vi "SCMP - darkflat.vi"(8 "error in (no error)":errorcluster, 10 "Dark/Flat":bool, 11 "Image Data Cluser":T1) -> (0 "error out":errorcluster, 2 "Raw Image Data2":u16[][](array[numeric]), 3 "Raw Image Data1":u16[][](array[numeric]), 4 "Y scale":i32, 6 "Image Data":u32[][](array[numeric]))   [LabVIEW 2014]
panel:
  out "dark/flat image":u32[][](graph)
  out "raw image":u32[][](graph)
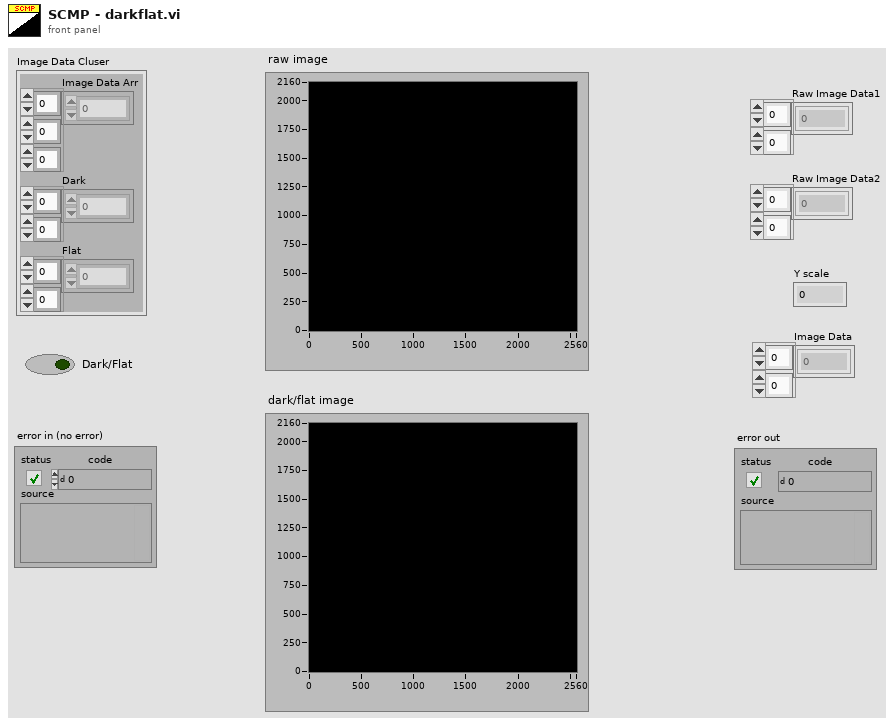
[diagram p1: front panel]
types:
  T1 = cluster{"Image Data Arr":u32[][][], "Dark":u32[][], "Flat":u32[][]}
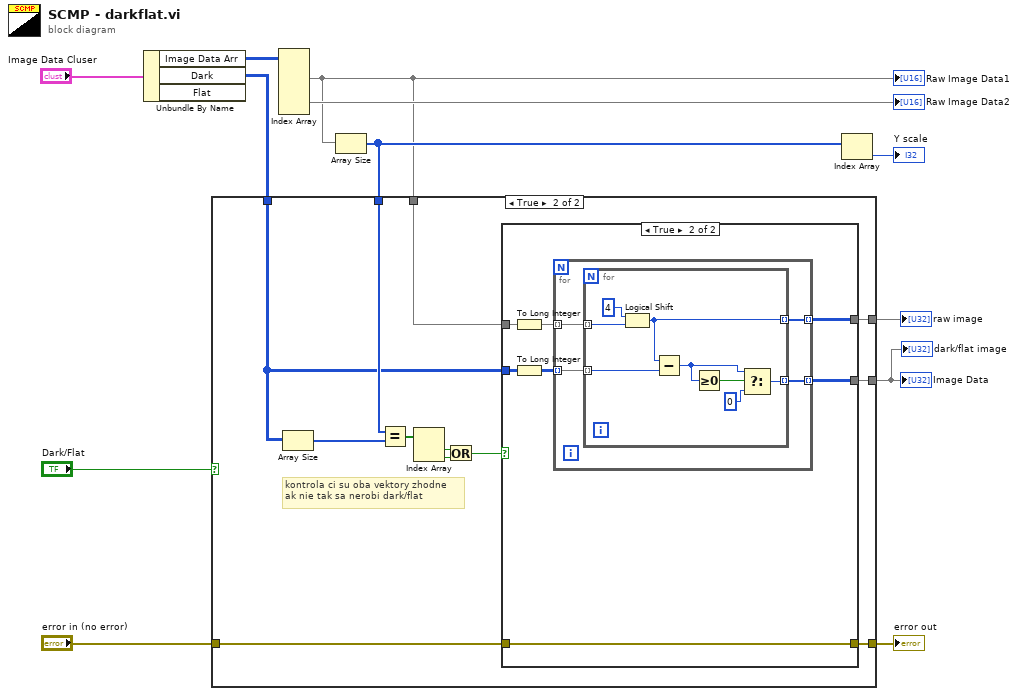
[diagram p0: block diagram]
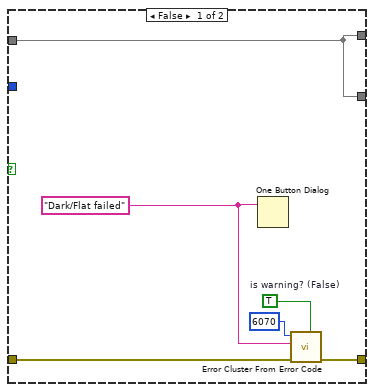
[diagram p3: hidden frame]
diagram:
  n1 = Unbundle By Name("Image Data Cluser") -> ("Image Data Arr"=w5:u32[][][], "Dark"=w4:u32[][])  [unwired: 1 out]
  n2 = Index Array(array=w5) -> (element #1=w3:u32[][], element #2=→"Raw Image Data2":u32[][])  [unwired: 6 in]
  "Raw Image Data1" <- w3
  n3 = Array Size(array=w3) -> (size(s)=w10:i32[])
  n4 = case shown="True" "Dark/Flat" {
    tunnel: w10 -> [_ w26]
    tunnel: "error in (no error)" -> [w14 w25]
    tunnel: [w14 w24] -> w8
    tunnel: w3 -> [w13 w18]
    tunnel: w4 -> [_ w17]
    tunnel: [w13 w16] -> w1
    tunnel: [w13 w15] -> w2
    frame False {
    }
    frame True {
      # "kontrola ci su oba vektory zhodne\nak nie tak sa nerobi dark/flat"
      n5 = Array Size(array=w17) -> (size(s)=w23:i32[])
      n6 = Equal?(x=w26, y=w23) -> (x = y?=w22:bool[])
      n7 = Index Array(array=w22) -> (element #1=w20:bool, element #2=w21:bool)  [unwired: 2 in]
      n8 = Or(x=w20, y=w21) -> (x .or. y?=w19:bool)
      n9 = case shown="True" w19 {
        tunnel: w25 -> [w32 w39]
        tunnel: [w31 w39] -> w24
        tunnel: w18 -> [w27 w38]
        tunnel: w17 -> [_ w37]
        tunnel: [w27 w34] -> w16
        tunnel: [w27 w33] -> w15
        frame False {
          w28 = "Dark/Flat failed" ("error message (\"\")")
          w30 = TRUE  # is warning? (False)
          n10 = One Button Dialog(message=w28) -> ()  [unwired: 1 in, 1 out]
          n11 = call <vilib>:"Error Cluster From Error Code.vi"("is warning? (False)"=w30, "error in (no error)"=w32, "error message (\"\")"=w28, "error code (0)"=6070) -> ("error out"=w31:errorcluster)  [unwired: 5 in]
        }
        frame True {
          n12 = To Long Integer(number=w38) -> (32bit integer=w36:i32[][])
          n13 = To Long Integer(number=w37) -> (32bit integer=w35:i32[][])
          n14 = for {
            tunnel: w36 -> [w43] mode=indexing
            tunnel: w35 -> [w42] mode=indexing
            tunnel: [w41] -> w34 mode=indexing
            tunnel: [w40] -> w33 mode=indexing
            n15 = for {
              tunnel: w43 -> [w50] mode=indexing
              tunnel: w42 -> [w49] mode=indexing
              tunnel: [w46] -> w41 mode=indexing
              tunnel: [w44] -> w40 mode=indexing
              n16 = Logical Shift(y=4 ("x"), x=w50) -> (x << y=w44:i32)
              n17 = Subtract(x=w44, y=w49) -> (x-y=w45:i32)
              n18 = Greater Or Equal To 0?(x=w45) -> (x >= 0?=w48:bool)
              n19 = Select(t=w45, s=w48, f=0) -> (s? t:f=w46:i32)
            }
          }
        }
      }
    }
  }
  "error out" <- w8
  "Image Data" <- w1
  "raw image" <- w2
  "dark/flat image" <- w1
  n20 = Index Array(array=w10) -> (element=→"Y scale":i32)  [unwired: 1 in]
